vi "color_image.vi"(9 "Blue Plane":u8[][](array[numeric]), 10 "Green Plane":u8[][](array[numeric]), 11 "Red plane":u8[][](array[numeric])) -> (3 "Color Image":T1)   [LabVIEW 2018]
uses:
  <vilib>/vision/Image Controls.llb/IMAQ Image.ctl
  <vilib>/vision/NI_Vision_Development_Module.lvlib
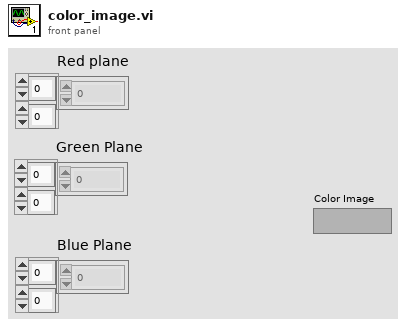
[diagram p1: front panel]
types:
  T1 = typedef "IMAQ Image.ctl" = refnum<image>
  T2 = typedef "Image Type" = u32
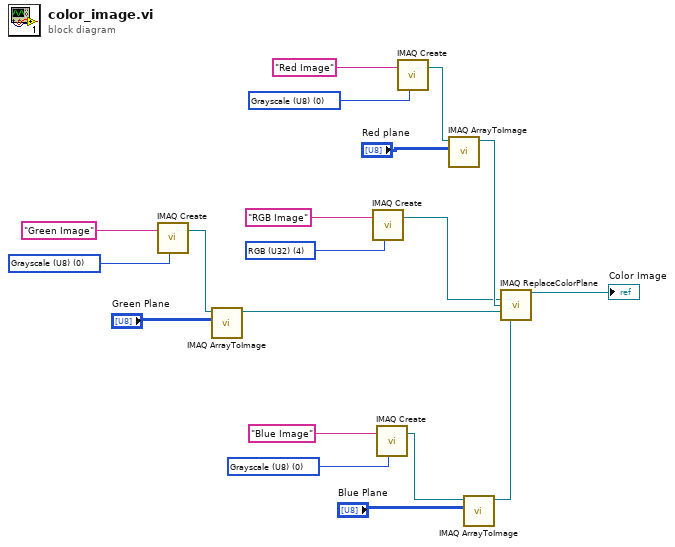
[diagram p0: block diagram]
diagram:
  w11 = T2 0 items=["Grayscale (U8)", "Grayscale (I16)", "Grayscale (SGL)", "Complex (CSG)", "RGB (U32)", "HSL (U32)", "RGB (U64)", "Grayscale (U16)"] ("Image Type")
  w13 = T2 0 items=["Grayscale (U8)", "Grayscale (I16)", "Grayscale (SGL)", "Complex (CSG)", "RGB (U32)", "HSL (U32)", "RGB (U64)", "Grayscale (U16)"] ("Image Type")
  w15 = T2 0 items=["Grayscale (U8)", "Grayscale (I16)", "Grayscale (SGL)", "Complex (CSG)", "RGB (U32)", "HSL (U32)", "RGB (U64)", "Grayscale (U16)"] ("Image Type")
  w18 = T2 4 items=["Grayscale (U8)", "Grayscale (I16)", "Grayscale (SGL)", "Complex (CSG)", "RGB (U32)", "HSL (U32)", "RGB (U64)", "Grayscale (U16)"] ("Image Type")
  n1 = call "IMAQ Create"("Image Name"="Green Image", "Image Type"=w13) -> ("New Image"=w9:T1)  [unwired: 3 in, 1 out]
  n2 = call "IMAQ ArrayToImage"("Image Pixels (U8)"="Green Plane", "Image"=w9) -> ("Image Out"=w6:T1)  [unwired: 8 in, 1 out]
  n3 = call "IMAQ Create"("Image Name"="RGB Image", "Image Type"=w18) -> ("New Image"=w4:T1)  [unwired: 3 in, 1 out]
  n4 = call "IMAQ Create"("Image Name"="Blue Image", "Image Type"=w11) -> ("New Image"=w8:T1)  [unwired: 3 in, 1 out]
  n5 = call "IMAQ Create"("Image Name"="Red Image", "Image Type"=w15) -> ("New Image"=w10:T1)  [unwired: 3 in, 1 out]
  n6 = call "IMAQ ArrayToImage"("Image Pixels (U8)"="Red plane", "Image"=w10) -> ("Image Out"=w7:T1)  [unwired: 8 in, 1 out]
  n7 = call "IMAQ ArrayToImage"("Image Pixels (U8)"="Blue Plane", "Image"=w8) -> ("Image Out"=w5:T1)  [unwired: 8 in, 1 out]
  n8 = call "IMAQ ReplaceColorPlane"("Image Dst"=w4, "Red or Hue Plane"=w7, "Green or Sat Plane"=w6, "Blue or Luma or Val or Inten Plane"=w5) -> ("Image Dst Out"=→"Color Image":T1)  [unwired: 10 in, 1 out]
